vi "Handle Response.vi"(7 "Processing In":refnum<class "Processing.lvclass">, 11 "Caching Response in":refnum<class "Caching Response.lvclass">) -> (0 "error out":errorcluster, 5 "Processing":refnum<class "Processing.lvclass">)   [LabVIEW 2023, in "HTTP Server.lvlib" / "Caching Response.lvclass"]
uses:
  Caching Response.lvclass
  Processing/Processing.lvclass
  Processing/Processing.lvclass/Processing.ctl
  lv-http-util/HTTP Utils/Request/Request.lvclass/Request.ctl
  Caching/Caching.lvclass
  C:/dev/volatus/mts-impulse/libs/lv-http-server/HTTP Server/Service/Service.lvclass
  lv-uri/URI/URI/URI.lvclass/URI.ctl
  lv-uri/URI/URI/Path String.vi
  lv-http-util/HTTP Utils/Request/Get Method.vi
  lv-http-util/HTTP Utils/Request/Request.lvclass
  lv-uri/URI/URI/URI.lvclass
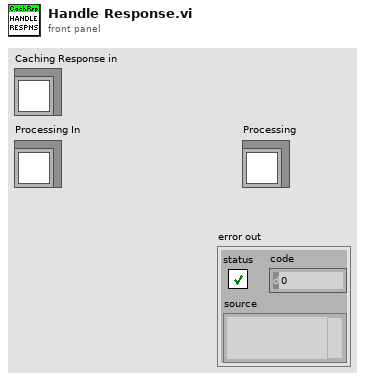
[diagram p1: front panel]
types:
  T1 = typedef "HTTP Utils.lvlib/Method.ctl" = enum16{"GET", "HEAD", "POST", "PUT", "DELETE", "CONNECT", "OPTIONS", "TRACE", "PATCH"}
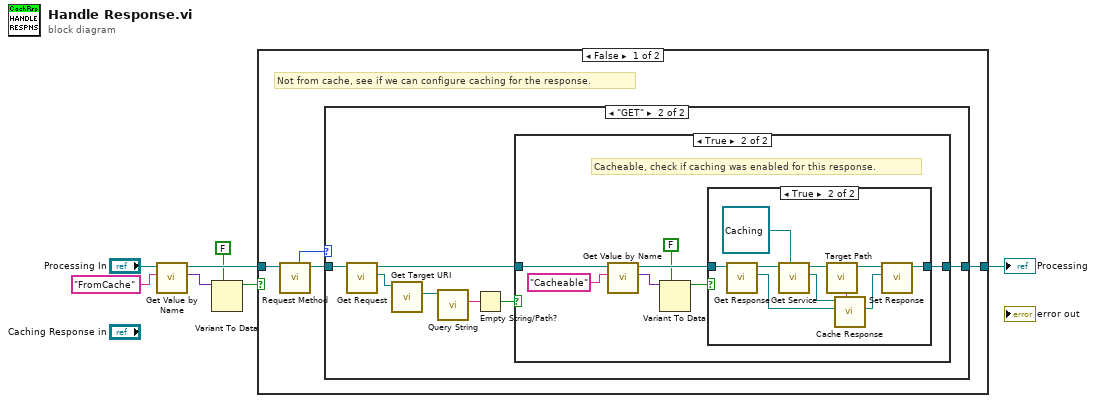
[diagram p0: block diagram]
diagram:
  n1 = call "Get Value by Name.vi"("Name"="FromCache" ("Name for Type"), "Processing in"="Processing In") -> ("Value"=w3:variant, "Processing out"=w5:refnum<class "Processing.lvclass">)  [unwired: 7 in, 1 out]
  n2 = Variant To Data(type=FALSE, Variant=w3) -> (data=w1:bool)  [unwired: 1 in, 1 out]
  n3 = case shown="False" w1 {
    tunnel: w5 -> [w11 w39]
    tunnel: [w8 w39] -> w4
    frame False {
      # "Not from cache, see if we can configure caching for the response."
      n4 = call "Request Method.vi"("Processing in"=w11) -> ("Processing out"=w9:refnum<class "Processing.lvclass">, "Request Method"=w10:T1)  [unwired: 9 in]
      n5 = case shown="\"GET\"" w10 {
        tunnel: w9 -> [w12 w19]
        tunnel: [w12 w13] -> w8
        frame Default {
          # "Only GET is cacheable."
        }
        frame "GET" {
          n6 = call "Get Request.vi"("Processing in"=w19) -> ("Request"=w18:refnum<class "Request.lvclass">, "Processing out"=w15:refnum<class "Processing.lvclass">)  [unwired: 9 in]
          n7 = call "Get Target URI.vi"("Request in"=w18) -> ("Target URI"=w17:refnum<class "URI.lvclass">)  [unwired: 8 in, 2 out]
          n8 = call "Query String.vi"("URI in"=w17) -> ("Query String"=w16:string)  [unwired: 9 in, 1 out]
          n9 = Empty String/Path?(string/path=w16) -> (empty?=w14:bool)
          n10 = case shown="True" w14 {
            tunnel: w15 -> [w20 w24]
            tunnel: [w20 w27] -> w13
            frame False {
              # "Don't cache when query is present."
            }
            frame True {
              # "Cacheable, check if caching was enabled for this response."
              n11 = call "Get Value by Name.vi"("Name"="Cacheable" ("Name for Type"), "Processing in"=w24) -> ("Value"=w23:variant, "Processing out"=w25:refnum<class "Processing.lvclass">)  [unwired: 7 in, 1 out]
              n12 = Variant To Data(type=FALSE, Variant=w23) -> (data=w22:bool)  [unwired: 1 in, 1 out]
              n13 = case shown="True" w22 {
                tunnel: w25 -> [w28 w33]
                tunnel: [w28 w35] -> w27
                frame False {
                }
                frame True {
                  n14 = call "Get Response.vi"("Processing in"=w33) -> ("Response"=w34:refnum<class "Response.lvclass">, "Processing out"=w32:refnum<class "Processing.lvclass">)  [unwired: 9 in]
                  n15 = call "Get Service.vi"("Service Type"=refnum<class "Caching.lvclass"> refnum ("HTTP Server.lvlib:Caching.lvclass"), "Processing in"=w32) -> ("Service"=w37:refnum<class "Caching.lvclass">, "Processing out"=w31:refnum<class "Processing.lvclass">)  [unwired: 7 in, 1 out]
                  n16 = call "Target Path.vi"("Processing in"=w31) -> ("Processing out"=w29:refnum<class "Processing.lvclass">, "Target Path"=w30:string)  [unwired: 9 in]
                  n17 = call "Cache Response.vi"("ID"=w30, "Response In"=w34, "Caching in"=w37) -> ("Response"=w36:refnum<class "Response.lvclass">)  [unwired: 7 in, 1 out]
                  n18 = call "Set Response.vi"("Response"=w36, "Processing in"=w29) -> ("Processing out"=w35:refnum<class "Processing.lvclass">)  [unwired: 9 in]
                }
              }
            }
          }
        }
      }
    }
    frame True {
      # "Was from cache, no need to do anything."
    }
  }
  "Processing" <- w4
